vi "Subvi DO.vi"(2 "DO channel":refnum<k21>="Connector1/DIO0", 10 "Memory label":refnum<k21>="DO0 buffer") -> ()   [LabVIEW 2017]
uses:
  <vilib>/rvi/Emulation/niFpgaGetClockAttributes.vi
  <vilib>/rvi/Emulation/niFpgaSctlEmulationGetInTimedLoop.vi
  <vilib>/rvi/Emulation/niFpgaEmulationReportErrorSimple.vi
  GV DO delay.vi
  <vilib>/rvi/DataTransferAndStorage/Container/Common/niFpgaContainerExecOnDevCompGetState.vi
  <vilib>/rvi/Emulation/niFpgaEmulationIsFPGAContextNoSignature.vi
  <vilib>/rvi/DataTransferAndStorage/Container/Common/niFpgaContainerGetUniqueNameForEmu.vi
  <vilib>/rvi/Emulation/niFpgaProcessEmulError.vi
  <vilib>/rvi/errors/nirviReportUnexpectedCaseInternalError (U32).vi
  <vilib>/rvi/Memory/Memory_Emulation/niFpgaMemoryEmulationCacheClearOnFirstRun.vi
  <vilib>/rvi/Memory/Memory_Emulation/nirvimemoryEmulationManagerCache_MakeExclusive.vi
  <vilib>/rvi/Memory/Memory_Emulation/niFpgaMemoryEmulationValidateCache.vi
  <vilib>/rvi/Memory/Memory_Emulation/nirvimemoryEmulationManagerCache_InsertValue.vi
  <vilib>/Utility/error.llb/Clear Errors.vi
  <vilib>/rvi/Memory/Memory_Emulation/nirvimemoryEmulationManagerCache_ReleaseExclusive.vi
  <vilib>/rvi/Memory/Memory_Emulation/nirvimemoryEmulationManagerCache_GetValue.vi
  <vilib>/rvi/Memory/Memory_Emulation/nirvimemoryEmulationManagerCache_SetValue.vi
  <vilib>/rvi/Emulation/niFpgaSctlEmulationResourceMgr.vi
  <vilib>/rvi/eio/common/nirviEmuTemplateMethod_errors.vi
  GV trigger.vi
  <vilib>/rvi/Emulation/niFpgaCriticalErrorInLSC.vi
  <vilib>/rvi/DataTransferAndStorage/Container/XNode/niFpgaContainer.xnode
  <vilib>/rvi/Memory/Memory_Emulation/niFpgaMemoryEmulationRefIn.vi
  <vilib>/eio/EIONode/EIONode.xnode
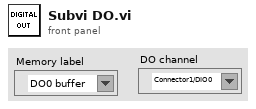
[diagram p1: front panel]
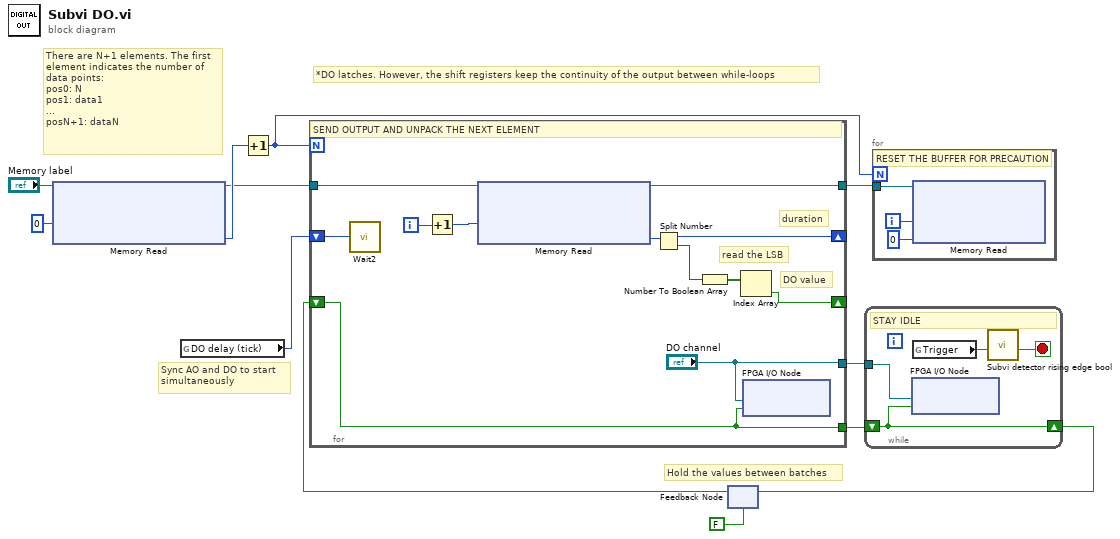
[diagram p0: block diagram]
diagram:
  # "There are N+1 elements. The first\nelement indicates the number of\ndata points:\npos0: N\npos1: data1\n...\nposN+1: dataN"
  # "Hold the values between batches"
  # "*DO latches. However, the shift registers keep the continuity of the output between while-loops"
  # "Sync AO and DO to start\nsimultaneously"
  n1 = xnode ("Memory Read")("Address"=u32 0, "Memory In"="Memory label") -> ("Data"=w4:u32, "Memory Out"=w1:refnum<k21>)
  n2 = global read "GV DO delay.vi" "DO delay (tick)"() -> (w12:u16)
  n3 = Increment(x=w4) -> (x+1=w3:u32)
  n4 = feedback #1(FALSE) -> (w8:bool)
  n5 = for {
    N: w3 -> [_]
    shift-right: [w18] -> _
    shift-left: w8 -> [w17]
    tunnel: [w17] -> w11
    shift-right: [w21] -> _
    shift-left: w12 -> [w20]
    tunnel: ["DO channel"] -> w10
    tunnel: [w16] -> w5
    tunnel: w1 -> [w15]
    i -> [w14]
    # "read the LSB"
    # "DO value"
    # "duration"
    # "SEND OUTPUT AND UNPACK THE NEXT ELEMENT"
    n6 = call "Wait2"("Count(Ticks)"=w20) -> ()  [unwired: 1 out]
    n7 = Increment(x=w14) -> (x+1=w13:i32)
    n8 = xnode ("Memory Read")("Address"=w13, "Memory In"=w15) -> ("Data"=w23:u32, "Memory Out"=w16:refnum<k21>)
    n9 = Split Number(x=w23) -> (hi(x)=w21:u16, lo(x)=w22:u16)
    n10 = Number To Boolean Array(number=w22) -> (Boolean array=w24:bool[])
    n11 = Index Array(array=w24) -> (element=w18:bool)  [unwired: 1 in]
    n12 = xnode "FPGA I/O Node"("I/O Item"=w17, "FPGA I/O In"="DO channel") -> ()  [unwired: 1 out]
  }
  n13 = while {
    shift-right: [w27] -> w9
    shift-left: w11 -> [w27]
    tunnel: w10 -> [w28]
    stop <- w25 stop-if-true
    # "STAY IDLE"
    n14 = xnode "FPGA I/O Node"("I/O Item"=w27, "FPGA I/O In"=w28) -> ()  [unwired: 1 out]
    n15 = global read "GV trigger.vi" "Trigger"() -> (w26:bool)
    n16 = call "Subvi detector rising edge bool.vi"("Input"=w26) -> ("Output"=w25:bool)  [unwired: 10 in]
  }
  n17 = feedback-in #1(w9) -> ()
  n18 = for {
    N: w3 -> [_]
    tunnel: w5 -> [w31]
    i -> [w30]
    # "RESET THE BUFFER FOR PRECAUTION"
    n19 = xnode ("Memory Read")("Address"=w30, "Data"=u32 0, "Memory In"=w31) -> ()  [unwired: 1 out]
  }
